vi "TopDown Field View.vi"(11 "XY":cluster{"X":dbl, "Y":dbl}) -> ()   [LabVIEW 2018]
panel:
  in  "Gyro":dbl
  out "Graph":cluster{cluster{"X":dbl, "Y":dbl}[]}[](graph)
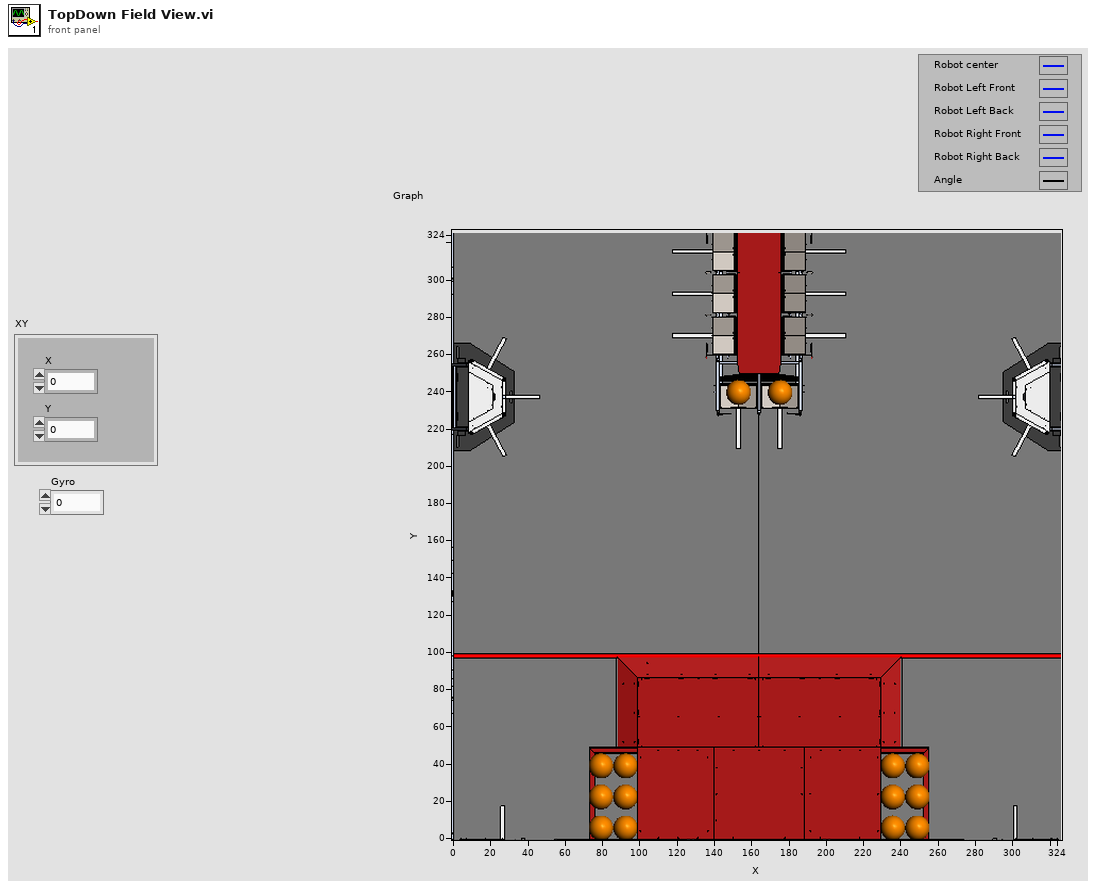
[diagram p1: front panel]
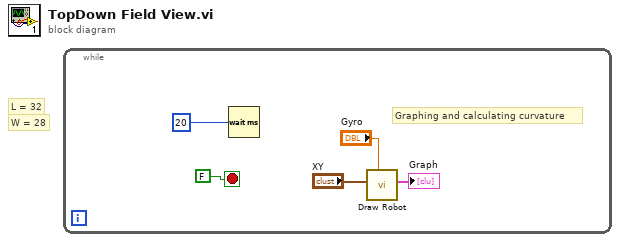
[diagram p0: block diagram]
diagram:
  # "W = 28"
  # "L = 32"
  n1 = while {
    stop <- FALSE stop-if-true
    # "Graphing and calculating curvature"
    n2 = Wait (ms)(milliseconds to wait=u32 20) -> ()  [unwired: 1 out]
    n3 = call "Draw Robot.vi"("Gyro"="Gyro", "XY"="XY") -> ("Graph 2"=→"Graph":cluster{cluster{"X":dbl, "Y":dbl}[]}[])  [unwired: 9 in]
  }
